vi "Directory Structure Example.vi"() -> ()   [LabVIEW 2024]
panel:
  out "String":string
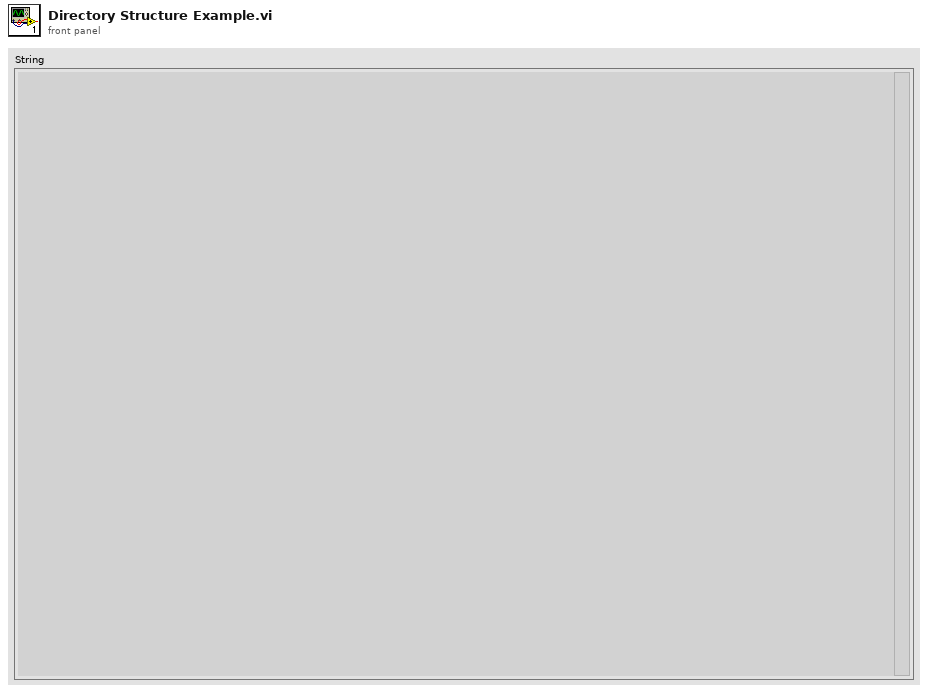
[diagram p1: front panel]
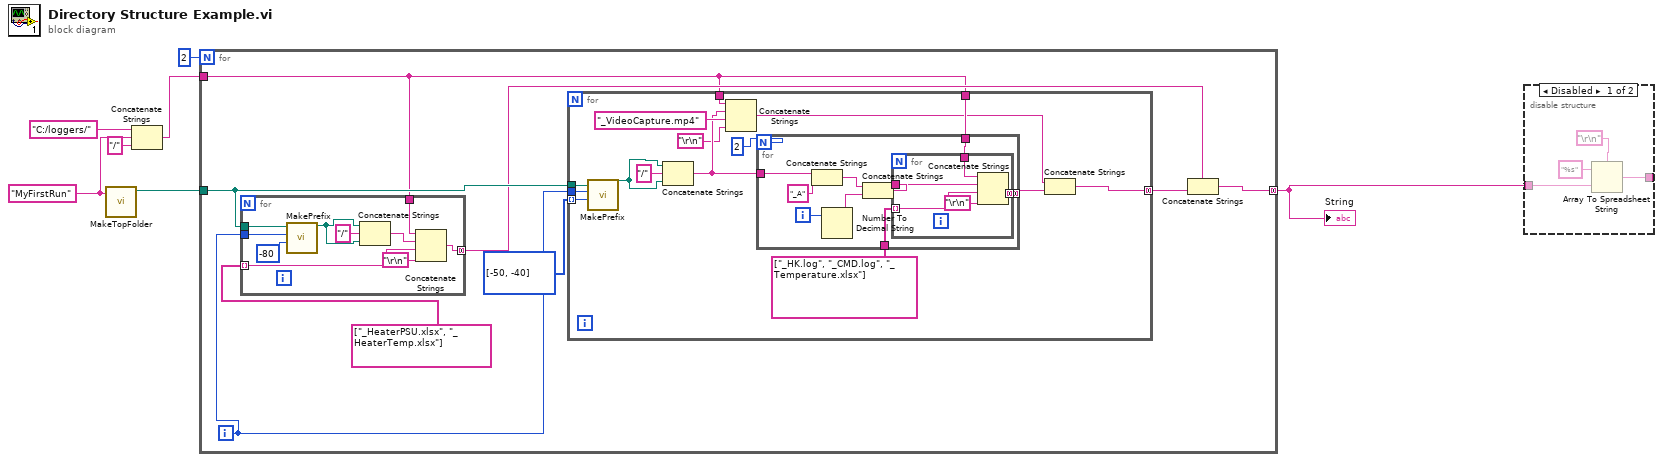
[diagram p0: block diagram]
diagram:
  w3 = "MyFirstRun" ("Comment")
  n1 = call "MakeTopFolder.vi"("Loggers"=w3) -> ("TestFolderPath"=w6:path)  [unwired: 9 in, 1 out]
  n2 = Concatenate Strings("C:/loggers/" ("string"), w3, "/" ("string")) -> (w1:string)
  n3 = for {
    N: 2 -> [_]
    tunnel: w6 -> [w12]
    tunnel: [w10] -> w7 mode=concatenating
    tunnel: w1 -> [w8]
    i -> [w11]
    n4 = for {
      tunnel: string[] ["_HeaterPSU.xlsx", "_HeaterTemp.xlsx"] -> [w25] mode=indexing
      tunnel: [w24] -> w9 mode=concatenating
      tunnel: w12 -> [w22]
      tunnel: w11 -> [w21]
      tunnel: w8 -> [w16]
      n5 = call "MakePrefix.vi"("TempCycleNo"=-80 ("TempPoint"), "FolderPrefix"=w21, "TopFolderPath"=w22) -> ("TestFolderPath"=w17:path)  [unwired: 7 in, 1 out]
      n6 = Concatenate Strings(w17, "/" ("string"), w17) -> (w19:string)
      n7 = Concatenate Strings(w16, w19, w25, "\r\n") -> (w24:string)
    }
    n8 = for {
      tunnel: i32[] [-50, -40] -> [w37] mode=indexing
      tunnel: w12 -> [w38]
      tunnel: [w28] -> w15 mode=concatenating
      tunnel: w11 -> [w33]
      tunnel: w8 -> [w32]
      tunnel: w8 -> [w26]
      n9 = call "MakePrefix.vi"("TempCycleNo"=w37, "FolderPrefix"=w33, "TopFolderPath"=w38) -> ("TestFolderPath"=w34:path)  [unwired: 7 in, 1 out]
      n10 = Concatenate Strings(w34, "/" ("string"), w34) -> (w30:string)
      n11 = Concatenate Strings(w26, w30, "_VideoCapture.mp4", "\r\n") -> (w27:string)
      n12 = for {
        N: 2 -> [_]
        tunnel: w30 -> [w47]
        tunnel: string[] ["_HK.log", "_CMD.log", "_Temperature.xlsx"] -> [w44]
        tunnel: [w42] -> w36 mode=concatenating
        tunnel: w32 -> [w41]
        i -> [w49]
        n13 = Concatenate Strings(w47, "_A" ("string")) -> (w46:string)
        n14 = Number To Decimal String(number=w49) -> (decimal integer string=w48:string)  [unwired: 1 in]
        n15 = Concatenate Strings(w46, w48) -> (w43:string)
        n16 = for {
          tunnel: w44 -> [w53] mode=indexing
          tunnel: w43 -> [w54]
          tunnel: [w52] -> w42 mode=concatenating
          tunnel: w41 -> [w50]
          n17 = Concatenate Strings(w50, w54, w53, "\r\n") -> (w52:string)
        }
      }
      n18 = Concatenate Strings(w27, w36) -> (w28:string)
    }
    n19 = Concatenate Strings(w9, w15) -> (w10:string)
  }
  "String" <- w7
  n20 = disable-structure shown="Disabled" {
    disable-tunnel: [w58 _] -> _
    disable-tunnel: w7 -> [w55 _]
    frame Disabled {
      n21 = Array To Spreadsheet String(delimiter (Tab)="\r\n", array=w55, 3:"%s" ("format string")) -> (spreadsheet string=w58:string)
    }
    frame Enabled {
    }
  }
